vi "produceTimingTicks.vi"(8 "error in (no error)":errorcluster, 10 "Channel":refnum<class "Channel.lvclass">, 11 "ScriptEventList in":refnum<class "ScriptEventList.lvclass">) -> (0 "error out":errorcluster, 2 "timingTickList":refnum<class "ScriptEventList.lvclass">, 3 "ScriptEventList out":refnum<class "ScriptEventList.lvclass">)   [LabVIEW 2009, in "Tools.lvlib" / "Scripting.lvlib" / "ScriptEventList.lvclass"]
uses:
  ScriptEventList.lvclass
  DatabaseHelpers/Database Objects/Channel/Channel.lvclass
  ScriptEventList.lvclass/ScriptEventList.ctl
  ScriptEvent.lvclass
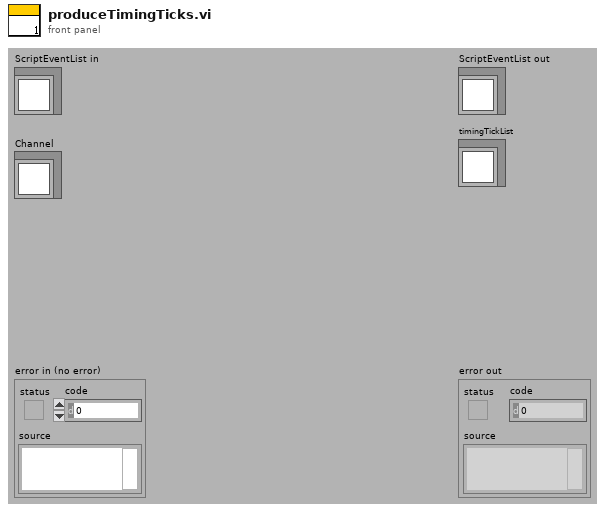
[diagram p1: front panel]
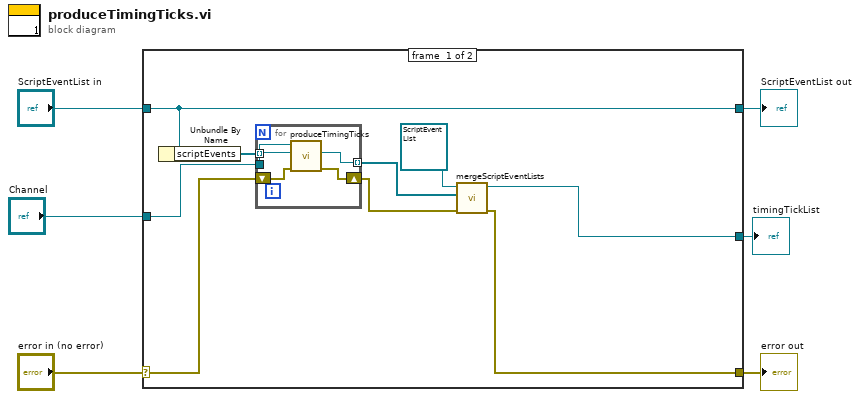
[diagram p0: block diagram]
diagram:
  n1 = case shown="No Error" "error in (no error)" {
    selector: "error in (no error)" -> [w13 w22]
    tunnel: [w7 w22] -> w5
    tunnel: [w15 w21] -> w3
    tunnel: "ScriptEventList in" -> [w15 w21]
    tunnel: [w9 _] -> w2
    tunnel: "Channel" -> [w12 _]
    frame #0 {
      n2 = Unbundle By Name(w15) -> ("scriptEvents"=w14:refnum<class "ScriptEvent.lvclass">[])
      n3 = for {
        tunnel: w14 -> [w20] mode=indexing
        shift-right: [w18] -> w8
        shift-left: w13 -> [w19]
        tunnel: [w17] -> w10 mode=indexing
        tunnel: w12 -> [w16]
        n4 = call-dynamic "produceTimingTicks.vi"("error in (no error)"=w19, "Channel"=w16, "ScriptEvent in"=w20) -> ("error out"=w18:errorcluster, "timingTick"=w17:refnum<class "ScriptEventList.lvclass">)  [unwired: 6 in, 1 out]
      }
      n5 = call "mergeScriptEventLists.vi"("error in (no error)"=w8, "Array"=w10, "ScriptEventList in"=refnum<class "ScriptEventList.lvclass"> refnum) -> ("error out"=w7:errorcluster, "ScriptEventList out"=w9:refnum<class "ScriptEventList.lvclass">)  [unwired: 7 in]
    }
    frame #1 {
    }
  }
  "error out" <- w5
  "ScriptEventList out" <- w3
  "timingTickList" <- w2
